vi "Resample Image.vi"(6 "Dest Binning":i32, 7 "Src Binning":i32, 8 "error in (no error)":errorcluster, 9 "Rescale Intensity? (F)":bool, 10 "Dest Image":T1, 11 "Src Image":T1) -> (0 "error out":errorcluster, 3 "Dest Image":T1)   [LabVIEW 2021, in "Image.lvlib"]
doc: "If <B>Dest Binning </B> or <Src Binnning</B> is <= 0, the <B>Src Image</B> is copied unchanged into <B>Dest Image</B>.\n\nThis VI uses <B>IMAQ Resample.vi</B> with the Bi-linear option for rescaling. \n\nIf <B>Rescale Intensity</B> is true, this VI rescales the data to emulate signal redistribution across pixels."
uses:
  Image.lvlib
  <vilib>/vision/Image Controls.llb/IMAQ Image.ctl
  <vilib>/vision/NI_Vision_Development_Module.lvlib
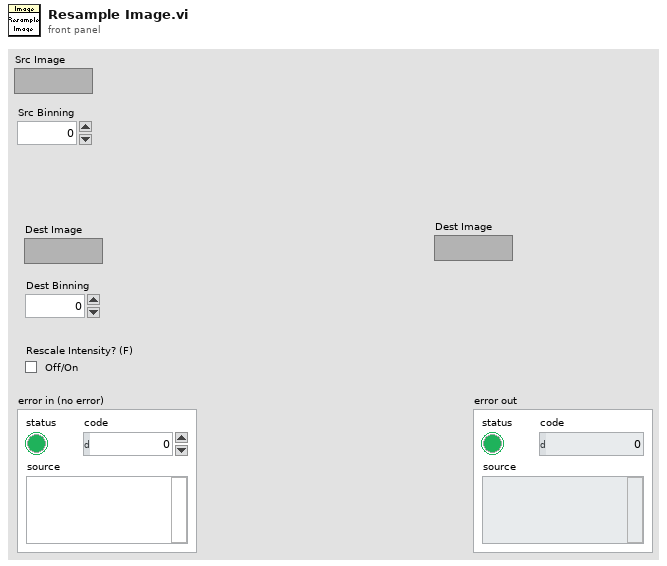
[diagram p1: front panel]
types:
  T1 = typedef "IMAQ Image.ctl" = refnum<image>
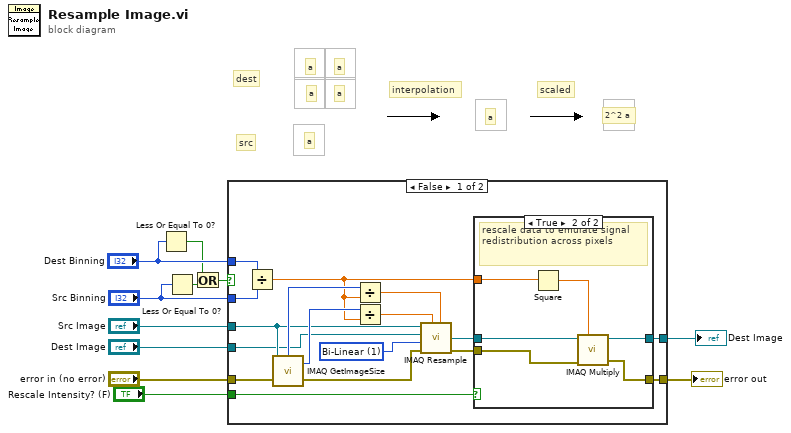
[diagram p0: block diagram]
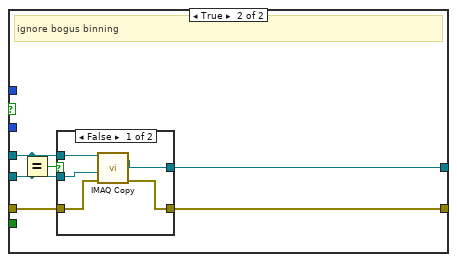
[diagram p3: hidden frame]
diagram:
  # "scaled"
  # "2^2 a"
  # "a"
  # "a"
  # "a"
  # "a"
  # "a"
  # "a"
  # "interpolation"
  # "src"
  # "dest"
  n1 = Less Or Equal To 0?(x="Dest Binning") -> (x <= 0?=w3:bool)
  n2 = Less Or Equal To 0?(x="Src Binning") -> (x <= 0?=w4:bool)
  n3 = Or(x=w3, y=w4) -> (x .or. y?=w2:bool)
  n4 = case shown="False" w2 {
    tunnel: [w18 w40] -> w11
    tunnel: "error in (no error)" -> [w25 w41]
    tunnel: [w19 w42] -> w9
    tunnel: "Src Image" -> [w24 w39]
    tunnel: "Dest Image" -> [w23 w38]
    tunnel: "Dest Binning" -> [w13 _]
    tunnel: "Src Binning" -> [w14 _]
    tunnel: "Rescale Intensity? (F)" -> [w22 _]
    frame False {
      w15 = u32 1 items=["Zero Order", "Bi-Linear", "Quadratic", "Cubic Spline"] ("Interpolation Type")
      n5 = Divide(x=w13, y=w14) -> (x/y=w12:dbl)
      n6 = call "IMAQ GetImageSize"("Image"=w24, "error in (no error)"=w25) -> ("Y Resolution"=w26:i32, "X Resolution"=w27:i32, "error out"=w28:errorcluster)  [unwired: 2 in]
      n7 = Divide(x=w27, y=w12) -> (x/y=w17:dbl)
      n8 = Divide(x=w26, y=w12) -> (x/y=w16:dbl)
      n9 = call "IMAQ Resample"("X Resolution"=w17, "Y Resolution"=w16, "error in (no error)"=w28, "Interpolation Type"=w15, "Image Dst"=w23, "Image Src"=w24) -> ("error out"=w20:errorcluster, "Image Dst Out"=w21:T1)  [unwired: 4 in]
      n10 = case shown="True" w22 {
        tunnel: w21 -> [w30 w36]
        tunnel: w20 -> [w29 w35]
        tunnel: [w30 w33] -> w19
        tunnel: [w29 w34] -> w18
        tunnel: w12 -> [_ w31]
        frame False {
        }
        frame True {
          # "rescale data to emulate signal redistribution across pixels"
          n11 = Square(x=w31) -> (x^2=w32:dbl)
          n12 = call "IMAQ Multiply"("Image Src A"=w36, "Constant"=w32, "error in (no error)"=w35) -> ("Image Dst Out"=w33:T1, "error out"=w34:errorcluster)  [unwired: 4 in]
        }
      }
    }
    frame True {
      # "ignore bogus binning"
      n13 = Equal?(x=w39, y=w38) -> (x = y?=w37:bool)
      n14 = case shown="False" w37 {
        tunnel: [w47 w48] -> w42
        tunnel: w41 -> [w46 w49]
        tunnel: [w45 w49] -> w40
        tunnel: w39 -> [w44 _]
        tunnel: w38 -> [w43 w48]
        frame False {
          n15 = call "IMAQ Copy"("error in (no error)"=w46, "Image Dst"=w43, "Image Src"=w44) -> ("error out"=w45:errorcluster, "Image Dst Out"=w47:T1)  [unwired: 3 in]
        }
        frame True {
        }
      }
    }
  }
  "error out" <- w11
  "Dest Image" <- w9
